vi "Log Action.vi"(10 "Log Packet":T1, 11 "Log Sink in":refnum<class "Log Sink.lvclass">) -> (0 "error out":errorcluster, 2 "Stop Sink?":bool, 3 "Log Sink out":refnum<class "Log Sink.lvclass">)   [LabVIEW 2020, in "Composed Log.lvlib" / "Log Sink.lvclass"]
uses:
  <vilib>/gpm_packages/@cs/event-logger/Source/Composed Log/Log Sink/Log Sink.lvclass
  <vilib>/gpm_packages/@cs/event-logger/Source/Composed Log/Types/Log Packet.ctl
  <vilib>/gpm_packages/@cs/event-logger/Source/Composed Log/Types/Log Level.ctl
  <vilib>/gpm_packages/@cs/event-logger/Source/Composed Log/Log Sink/Log Sink.lvclass/Log Sink.ctl
  <vilib>/gpm_packages/@cs/event-logger/Source/Composed Log/Log Sink/Check Should Log.vi
  <vilib>/gpm_packages/@cs/event-logger/Source/Composed Log/ILogFilter/ILogFilter.lvclass
  <vilib>/gpm_packages/@cs/event-logger/Source/Composed Log/Composed Log.lvlib
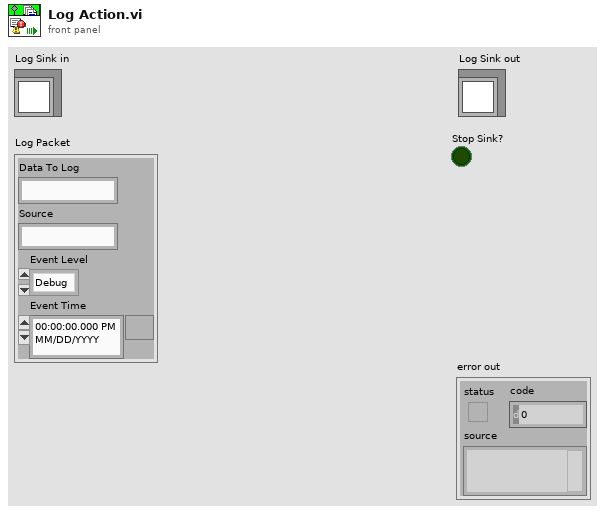
[diagram p1: front panel]
types:
  T1 = typedef "Composed Log.lvlib/Log Packet.ctl" = cluster{"Data To Log":string, "Source":string, "Event Level":T2, "Event Time":timestamp}
  T2 = typedef "Composed Log.lvlib/Log Level.ctl" = enum16{"Debug", "Info", "Warning", "Error", "Critical"}
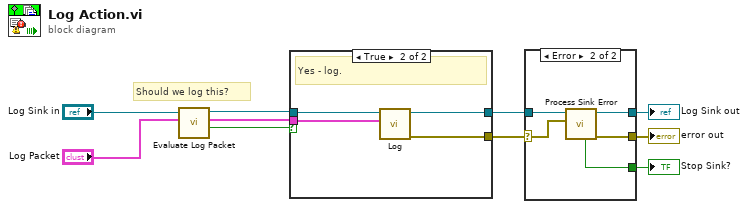
[diagram p0: block diagram]
diagram:
  # "Should we log this?"
  n1 = call <vilib>:"Evaluate Log Packet.vi"("Log Packet"="Log Packet", "Log Sink in"="Log Sink in") -> ("Log?"=w3:bool, "Log Packet Out"=w4:T1, "Log Sink out"=w5:refnum<class "Log Sink.lvclass">)  [unwired: 7 in]
  n2 = case shown="True" w3 {
    tunnel: w5 -> [w11 w14]
    tunnel: [w11 w15] -> w9
    tunnel: w4 -> [_ w13]
    tunnel: [_ w12] -> w10
    frame False {
      # "Nope - just ignore."
    }
    frame True {
      # "Yes - log."
      n3 = call-dynamic "Log.vi"("Log Packet"=w13, "Log Sink in"=w14) -> ("error out"=w12:errorcluster, "Log Sink out"=w15:refnum<class "Log Sink.lvclass">)  [unwired: 8 in]
    }
  }
  n4 = case shown="Error" w10 {
    selector: w10 -> [w16 w19]
    tunnel: w9 -> [w17 w22]
    tunnel: [w17 w21] -> w8
    tunnel: [w16 w20] -> w7
    tunnel: [_ w18] -> w2
    frame No Error {
    }
    frame Error {
      n5 = call-dynamic "Process Sink Error.vi"("Error To Process"=w19, "Log Sink in"=w22) -> ("error out"=w20:errorcluster, "Log Sink out"=w21:refnum<class "Log Sink.lvclass">, "Stop Sink?"=w18:bool)  [unwired: 7 in]
    }
  }
  "error out" <- w7
  "Log Sink out" <- w8
  "Stop Sink?" <- w2
